vi "Main.vi"() -> ()   [LabVIEW 2014]
panel:
  out "경로":path
  out "웨이브폼 그래프":dbl[](graph)
  in  "정지":bool
  in  "Sub VI":bool
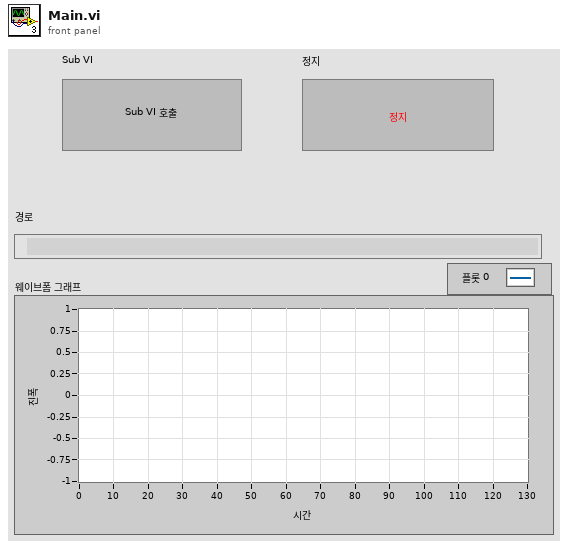
[diagram p1: front panel]
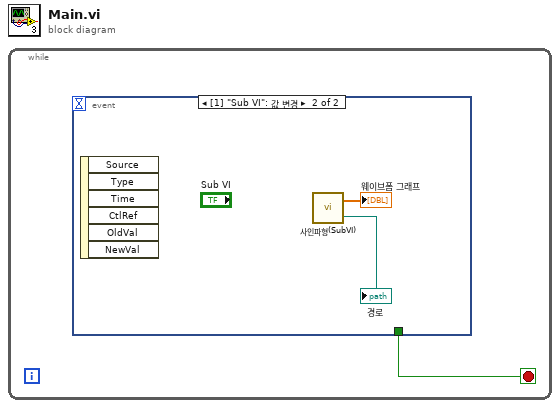
[diagram p0: block diagram]
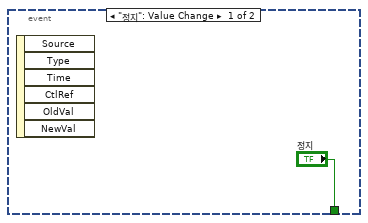
[diagram p2: hidden frame]
diagram:
  n1 = while {
    stop <- w1 stop-if-true
    n2 = event shown="[1] \"Sub VI\": 값 변경" {
      selector: _ -> [_ _]
      dyn-events: _ -> [_ _]
      timeout: _ -> [_ _]
      tunnel: ["정지" _] -> w1
      event "정지": Value Change {
        n3 = event-data() -> ()  [unwired: 1 in, 6 out]
      }
      event "Sub VI": Value Change {
        n4 = event-data() -> ()  [unwired: 1 in, 6 out]
        n5 = call "사인파형(SubVI).vi"() -> ("경로"=→"경로":path, "웨이브폼 그래프"=→"웨이브폼 그래프":dbl[])  [unwired: 2 in]
      }
    }
  }
